vi "DegreetoSpeed.vi"(10 "Command":i8, 11 "Torque":dbl) -> (3 "Numeric":dbl)   [LabVIEW 2018]
panel:
  out "concatenated string":string
  out "resulting string 2":string
  out "resulting string":string
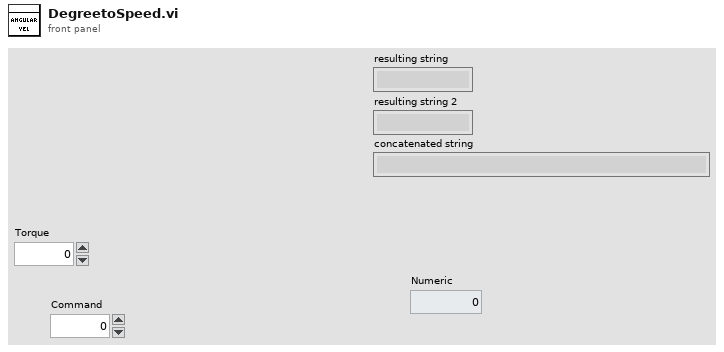
[diagram p1: front panel]
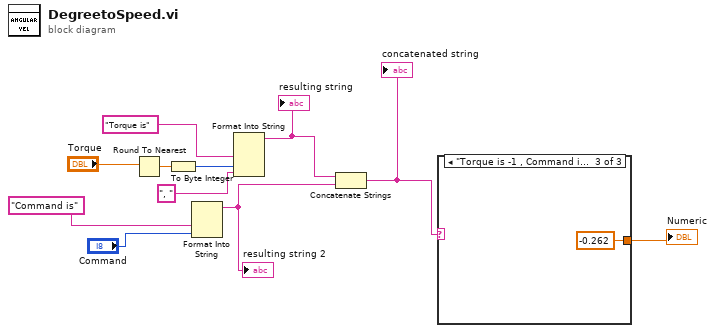
[diagram p0: block diagram]
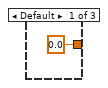
[diagram p2: hidden frame]
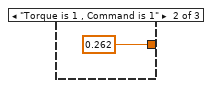
[diagram p3: hidden frame]
diagram:
  n1 = Round To Nearest(number="Torque") -> (nearest integer value=w6:dbl)
  n2 = To Byte Integer(number=w6) -> (8bit integer=w5:i8)
  n3 = Format Into String("Command is", "Command") -> (resulting string=w9:string)  [unwired: 3 in, 1 out]
  "resulting string 2" <- w9
  n4 = Format Into String("Torque is", w5, ", ") -> (resulting string=w10:string)  [unwired: 3 in, 1 out]
  "resulting string" <- w10
  n5 = Concatenate Strings(w10, w9) -> (w8:string)
  "concatenated string" <- w8
  n6 = case shown="\"Torque is -1 , Command is 0\"" w8 {
    tunnel: [0.0 0.262 -0.262] -> w1
    frame Default {
    }
    frame "Torque is 1 , Command is 1" {
    }
    frame "Torque is -1 , Command is 0" {
    }
  }
  "Numeric" <- w1
